vi "PQ Example COPY file.vi"() -> ()   [LabVIEW 2016]
uses:
  Connection/PQ Connection.lvclass
panel:
  out "Copy Rate (MB/s)":dbl
  in  "table name":string
  in  "connection string":string
  out "Copy Time (s)":dbl
  out "buffer":string
  in  "File":path
  out "error out":errorcluster
  # "Read connection info from PGPASS file if this field is blank:"
  # "Table name on database to copy to:"
  # "Spreadsheet file with header that matches target table:"
  # "data to write:"
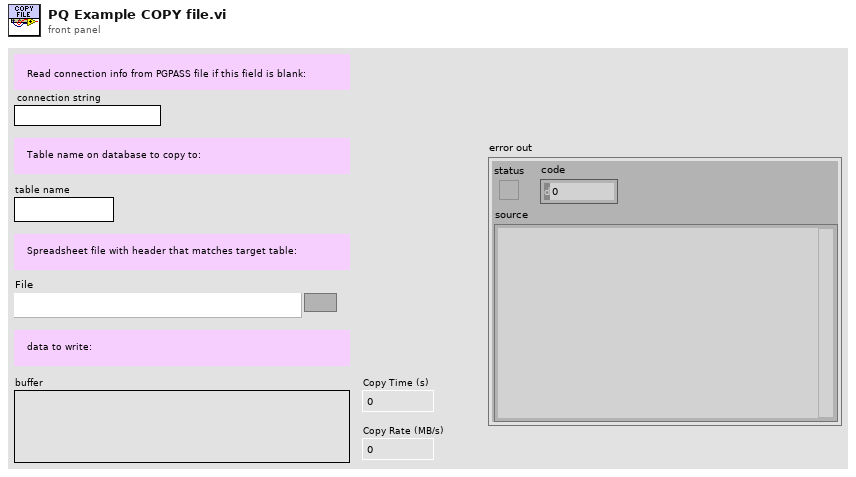
[diagram p1: front panel]
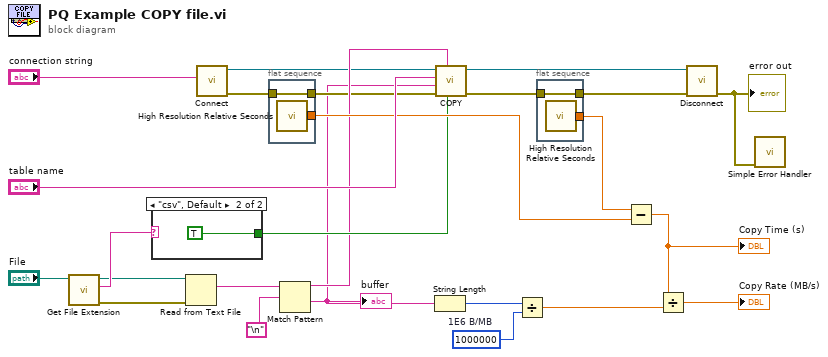
[diagram p0: block diagram]
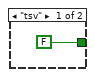
[diagram p2: hidden frame]
diagram:
  w2 = 1000000  # 1E6 B/MB
  n1 = call <vilib>:"Get File Extension.vi"("file"="File") -> ("error out"=w13:errorcluster, "lowercase file extension"=w18:string, "dup file"=w14:path)  [unwired: 6 in, 2 out]
  n2 = case shown="\"csv\", Default" w18 {
    tunnel: [FALSE TRUE] -> w17
    frame "tsv" {
    }
    frame "csv", Default {
    }
  }
  n3 = Read from Text File(file (use dialog)=w14, error in=w13) -> (text=w20:string)  [unwired: 2 in, 3 out]
  n4 = call "Connect.vi"("Connection Strings"="connection string") -> ("error out"=w12:errorcluster, "PQ Connection out"=w9:refnum<class "PQ Connection.lvclass">)  [unwired: 9 in]
  n5 = flat-sequence {
    tunnel: w12 -> [w29]
    tunnel: [w29] -> w7
    tunnel: [w28] -> w21
    frame #0 {
      n6 = call <vilib>:"High Resolution Relative Seconds.vi"() -> ("relative seconds"=w28:dbl)
    }
  }
  n7 = Match Pattern(string=w20, regular expression="\n") -> (before substring=w16:string, after substring=w6:string)  [unwired: 1 in, 2 out]
  "buffer" <- w6
  n8 = String Length(string=w6) -> (length=w5:i32)
  n9 = call "COPY.vi"("CSV?"=w17, "column name(s) (empty=ALL)"=w16, "error in (no error)"=w7, "buffer"=w6, "table name"="table name", "PQ Connection in"=w9) -> ("error out"=w10:errorcluster, "PQ Connection out"=w8:refnum<class "PQ Connection.lvclass">)  [unwired: 4 in]
  n10 = Divide(x=w5, y=w2) -> (x/y=w4:dbl)
  n11 = flat-sequence {
    tunnel: w10 -> [w31]
    tunnel: [w31] -> w11
    tunnel: [w30] -> w23
    frame #0 {
      n12 = call <vilib>:"High Resolution Relative Seconds.vi"() -> ("relative seconds"=w30:dbl)
    }
  }
  n13 = Subtract(x=w23, y=w21) -> (x-y=w1:dbl)
  "Copy Time (s)" <- w1
  n14 = Divide(x=w1, y=w4) -> (x/y=→"Copy Rate (MB/s)":dbl)
  n15 = call-dynamic "Disconnect.vi"("error in (no error)"=w11, "PQ Connection in"=w8) -> ("error out"=w25:errorcluster)  [unwired: 9 in]
  "error out" <- w25
  n16 = call <vilib>:"Simple Error Handler.vi"("error in (no error)"=w25) -> ()  [unwired: 4 in, 5 out]
